vi "Exemple_Preprocessing_LabelBinarizer.vi"() -> ()   [LabVIEW 2020]
uses:
  Objet/6 - Datasets Transformation/6.3 - Processing Data/LabelBinarizer/LabelBinarizer.lvclass
panel:
  in  "y":string[][](array[string])=[["1"], ["2"], ["6"], ["4"], ["2"]]
  out "Data":T1
  out "error out":errorcluster
  in  "error in":errorcluster caption="entrée d'erreur"
  in  "LabelBinarizer":T2={"neg_label"=0, "pos_label"=1, "sparse_output"=FALSE}
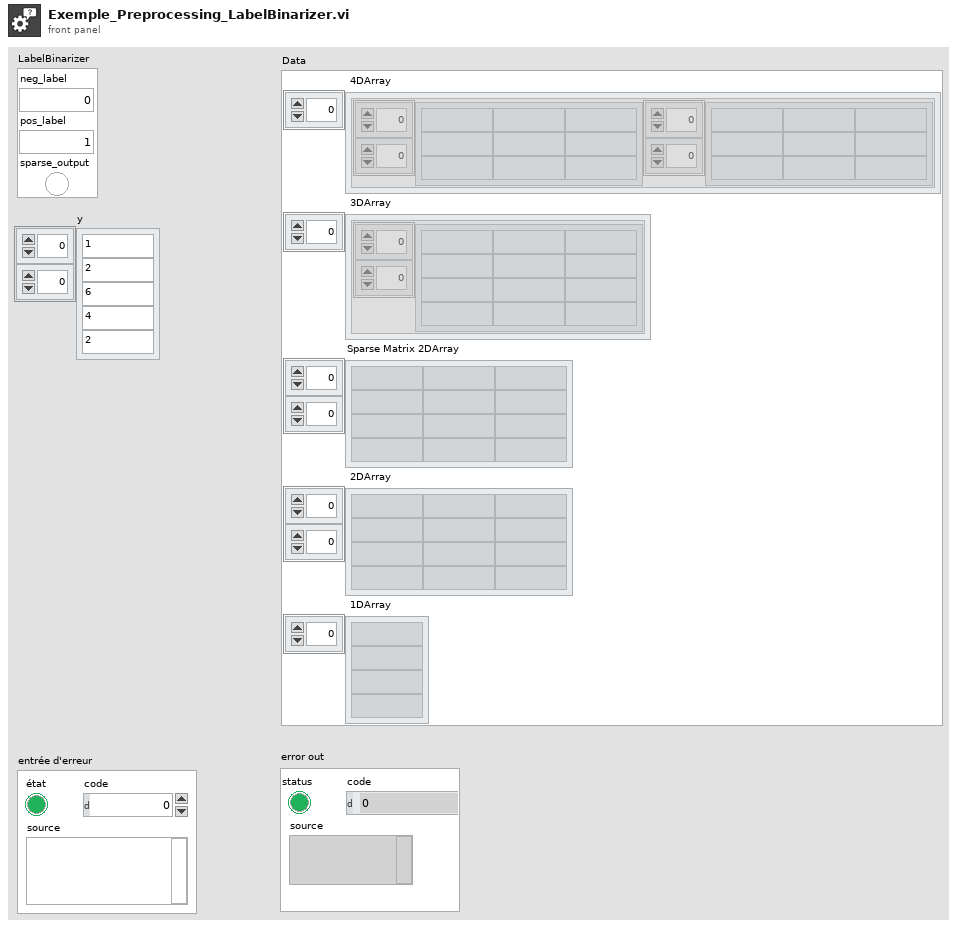
[diagram p1: front panel]
types:
  T1 = cluster{" 4DArray":cluster{"1":string[][], "2":string[][]}[], " 3DArray":cluster{"Tableau":string[][]}[], "Sparse Matrix 2DArray":string[][], " 2DArray":string[][], " 1DArray":string[]}
  T2 = cluster{"neg_label":i32, "pos_label":i32, "sparse_output":bool}
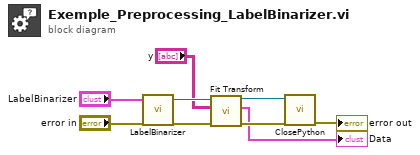
[diagram p0: block diagram]
diagram:
  n1 = call "LabelBinarizer.vi"("error in (no error)"="error in", "LabelBinarizer"="LabelBinarizer") -> ("error out"=w8:errorcluster, "LabelBinarizer.lvclass"=w9:refnum<class "LabelBinarizer.lvclass">)  [unwired: 8 in]
  n2 = call-dynamic "Fit Transform.vi"("error in (no error)"=w8, "y"="y", "LabelBinarizer.lvclass"=w9) -> ("error out"=w7:errorcluster, "Data"=→"Data":T1, "LabelBinarizer.lvclass"=w6:refnum<class "LabelBinarizer.lvclass">)  [unwired: 6 in]
  n3 = call-dynamic "ClosePython.vi"("error in (no error)"=w7, "Scikit-learn en entrée"=w6) -> ("error out"=→"error out":errorcluster)  [unwired: 8 in, 1 out]
